vi "Message.vi"(8 "error in (no error)":errorcluster, 9 "Additional text":string, 10 "Message":T1) -> (0 "error out":errorcluster)   [LabVIEW 2013, in "SettingsFile.lvlib" / "SettingsFile.lvclass"]
uses:
  SettingsFile.lvclass
  Messages.ctl
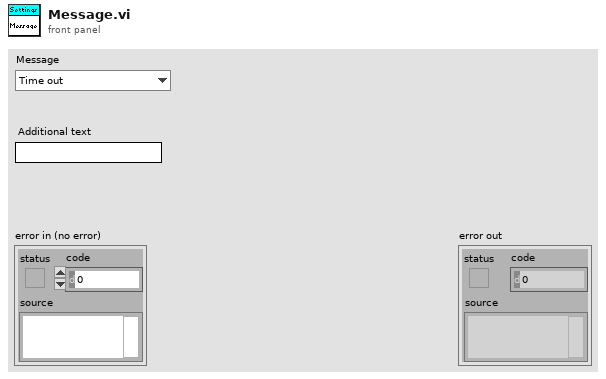
[diagram p1: front panel]
types:
  T1 = typedef "SettingsFile.lvlib/SettingsFile.lvclass/Messages.ctl" = enum16{"Time out", "User cancel", "Module cancel", "File format change"}
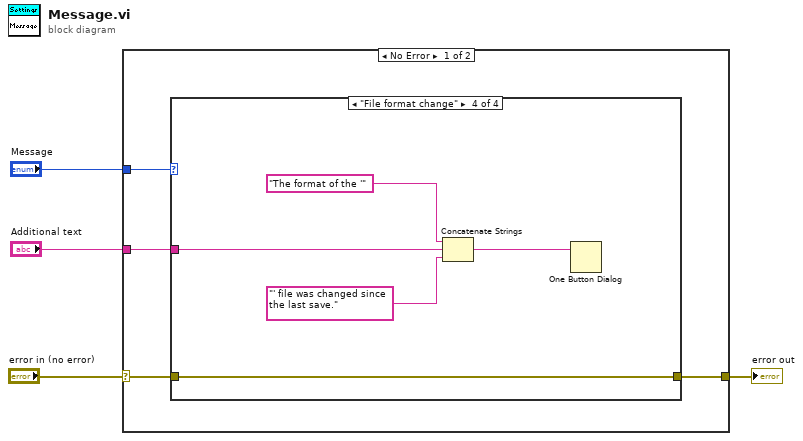
[diagram p0: block diagram]
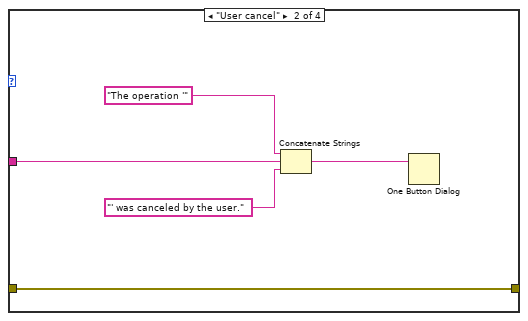
[diagram p3: hidden frame]
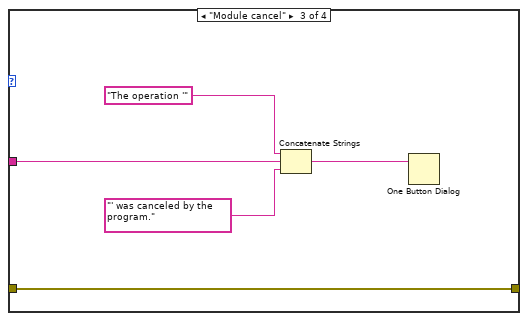
[diagram p4: hidden frame]
diagram:
  n1 = case shown="No Error" "error in (no error)" {
    selector: "error in (no error)" -> [w8 w25]
    tunnel: [w5 w25] -> w3
    tunnel: "Message" -> [w7 _]
    tunnel: "Additional text" -> [w6 _]
    frame No Error {
      n2 = case shown="\"File format change\"" w7 {
        tunnel: w8 -> [w9 w14 w19 w24]
        tunnel: w6 -> [_ w13 w18 w23]
        tunnel: [w9 w14 w19 w24] -> w5
        frame Default {
        }
        frame "User cancel" {
          n3 = Concatenate Strings("The operation '", w13, "' was canceled by the user.") -> (w10:string)
          n4 = One Button Dialog(message=w10) -> ()  [unwired: 1 in, 1 out]
        }
        frame "Module cancel" {
          n5 = Concatenate Strings("The operation '", w18, "' was canceled by the program.") -> (w15:string)
          n6 = One Button Dialog(message=w15) -> ()  [unwired: 1 in, 1 out]
        }
        frame "File format change" {
          n7 = Concatenate Strings("The format of the '", w23, "' file was changed since the last save.") -> (w20:string)
          n8 = One Button Dialog(message=w20) -> ()  [unwired: 1 in, 1 out]
        }
      }
    }
    frame Error {
    }
  }
  "error out" <- w3
